vi "Configure Sequence (Pulse).vi"(0 "VISA resource name":refnum<visa-resource-name>, 1 "Channel Name (1)":string="1", 3 "Pulse Sequence Width (1.0 s)":dbl=1.0 format="%^.3e", 4 "Waveform Type (1: Voltage)":i32(ring)=1 items=["Voltage"=1, "Current"=0], 5 "error in (no error)":errorcluster {"code" format="%.0x"}, 6 "Pulse Sequence Start Time (0.0 s)":dbl format="%^.3e", 7 "Pulse Sequence End Time (0.0 s)":dbl format="%^.3e", 8 "Pulse Sequence Start Level (0.0)":dbl format="%^.3e", 9 "Pulse Sequence Amplitude (0.0)":dbl format="%^.3e", 12 "Sequence Step Number (0)":i32) -> (14 "VISA resource name out":refnum<visa-resource-name>, 19 "error out":errorcluster {"code" format="%.0x"})   [LabVIEW 2018, in "Agilent N6700 Series.lvlib"]
doc: "Configures the pulse sequence.\n\n<b>Note:</b>\nThis VI only applies to the N6705B and N6705C DC Power Analyzer."
uses:
  Agilent N6700 Series.lvlib
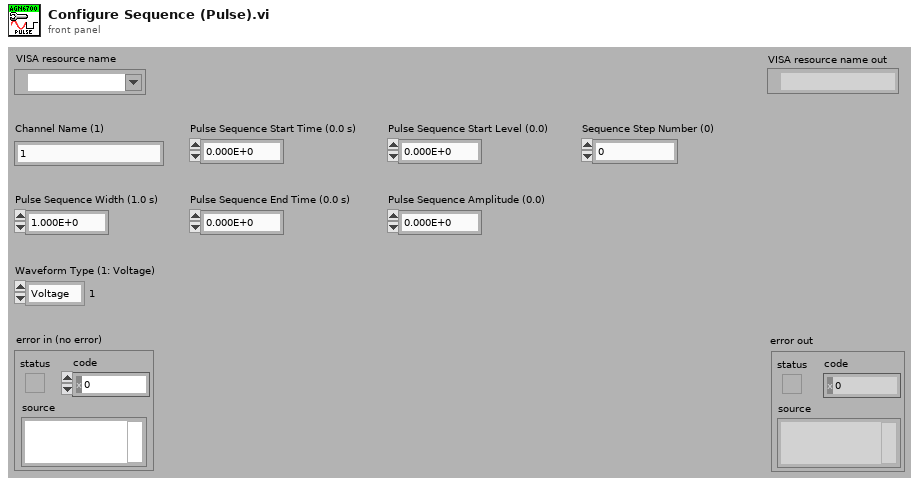
[diagram p1: front panel]
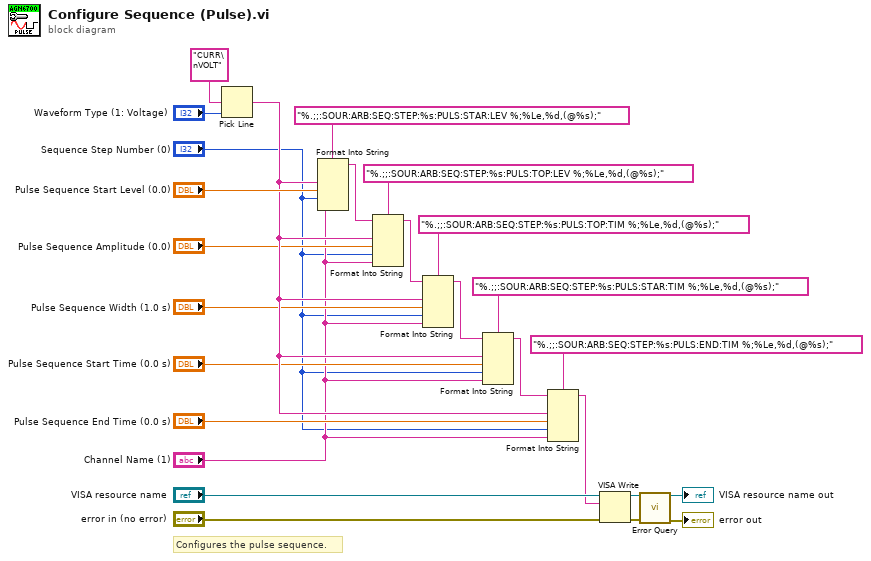
[diagram p0: block diagram]
diagram:
  # "Configures the pulse sequence."
  n1 = Pick Line(multi-line string="CURR\nVOLT", line index="Waveform Type (1: Voltage)") -> (output string=w11:string)  [unwired: 1 in]
  n2 = Format Into String(format string="%.;;:SOUR:ARB:SEQ:STEP:%s:PULS:STAR:LEV %;%Le,%d,(@%s);", w11, "Pulse Sequence Start Level (0.0)", "Sequence Step Number (0)", "Channel Name (1)") -> (resulting string=w16:string)  [unwired: 2 in, 1 out]
  n3 = Format Into String(format string="%.;;:SOUR:ARB:SEQ:STEP:%s:PULS:TOP:LEV %;%Le,%d,(@%s);", initial string=w16, w11, "Pulse Sequence Amplitude (0.0)", "Sequence Step Number (0)", "Channel Name (1)") -> (resulting string=w15:string)  [unwired: 1 in, 1 out]
  n4 = Format Into String(format string="%.;;:SOUR:ARB:SEQ:STEP:%s:PULS:TOP:TIM %;%Le,%d,(@%s);", initial string=w15, w11, "Pulse Sequence Width (1.0 s)", "Sequence Step Number (0)", "Channel Name (1)") -> (resulting string=w14:string)  [unwired: 1 in, 1 out]
  n5 = Format Into String(format string="%.;;:SOUR:ARB:SEQ:STEP:%s:PULS:STAR:TIM %;%Le,%d,(@%s);", initial string=w14, w11, "Pulse Sequence Start Time (0.0 s)", "Sequence Step Number (0)", "Channel Name (1)") -> (resulting string=w13:string)  [unwired: 1 in, 1 out]
  n6 = Format Into String(format string="%.;;:SOUR:ARB:SEQ:STEP:%s:PULS:END:TIM %;%Le,%d,(@%s);", initial string=w13, w11, "Pulse Sequence End Time (0.0 s)", "Sequence Step Number (0)", "Channel Name (1)") -> (resulting string=w12:string)  [unwired: 1 in, 1 out]
  n7 = VISA Write(VISA resource name="VISA resource name", write buffer=w12, error in (no error)="error in (no error)") -> (VISA resource name out=w22:refnum<visa-resource-name>, error out=w21:errorcluster)  [unwired: 1 out]
  n8 = call "Error Query.vi"("VISA resource name"=w22, "error in (no error)"=w21) -> ("VISA resource name out"=→"VISA resource name out":refnum<visa-resource-name>, "error out"=→"error out":errorcluster)  [unwired: 10 in, 2 out]
